vi "LiftMain.vi"(6 "Lift Override":bool, 8 "Error In":errorcluster, 9 "Reverse":bool, 10 "Forward":bool, 11 "Control Mode":enum16{"Open", "Control"}(ring)) -> (0 "Error Out":errorcluster, 2 "Switch Pressed":bool)   [LabVIEW 2016]
uses:
  <vilib>/Rock Robotics/SystemInterfaces/DIO/FPGA_DIORelayChannel.ctl
  <vilib>/Rock Robotics/WPI/Relay/WPI_RelayDirection.ctl
  <vilib>/Rock Robotics/SystemInterfaces/DIO/FPGA_DIOChannel.ctl
  <vilib>/Rock Robotics/WPI/Relay/WPI_RelayValue.ctl
  <vilib>/Rock Robotics/WPI/Switch/WPI_SwitchOpenLimit.vi
  <vilib>/Rock Robotics/Network Tables/NT Read Number.vi
panel:
  # "Lift Control Main VI\nFRC Team 34"
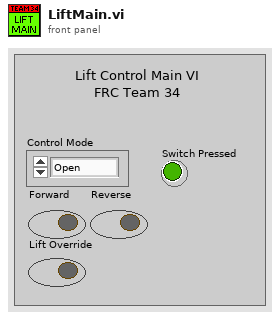
[diagram p1: front panel]
types:
  T1 = typedef "FPGA_DIOChannel.ctl" = enum8{"DIO 0", "DIO 1", "DIO 2", "DIO 3", "DIO 4", "DIO 5", "DIO 6", "DIO 7", "DIO 8", "DIO 9", "DIO MXP 0", "DIO MXP 1", "DIO MXP 2", "DIO MXP 3", "DIO MXP 4", "DIO MXP 5", "DIO MXP 6", "DIO MXP 7", "DIO MXP 8", "DIO MXP 9", "DIO MXP 10", "DIO MXP 11", "DIO MXP 12", "DIO MXP 13", "DIO MXP 14", "DIO MXP 15", "SPI Port CS1", "SPI Port CS2", "SPI Port CS3", "SPI Port MISO", "SPI Port MOSI", "Invalid"}
  T2 = typedef "WPI_RelayDirection.ctl" = enum16{"Both directions", "Forward only", "Reverse only"}
  T3 = typedef "FPGA_DIORelayChannel.ctl" = enum8{"Relay 0", "Relay 1", "Relay 2", "Relay 3", "Invalid"}
  T4 = typedef "WPI_RelayValue.ctl" = enum16{"Off", "On", "Forward", "Reverse"}
  T5 = typedef "WPI_SwitchDevRef.ctl" = cluster{"DevStatus":errorcluster, "DIO Channel":T1, "CntIndex":T6, "Normally Closed":bool}
  T6 = typedef "FPGA_CounterCtrSystemIndex.ctl" = enum8{"Ctr 0", "Ctr 1", "Ctr 2", "Ctr 3", "Ctr 4", "Ctr 5", "Ctr 6", "Ctr 7", "Invalid"}
  T7 = typedef "WPI_RelayDevRef.ctl" = cluster{"DevStatus":errorcluster, "Relay Channel":T3, "Relay Direction":T2}
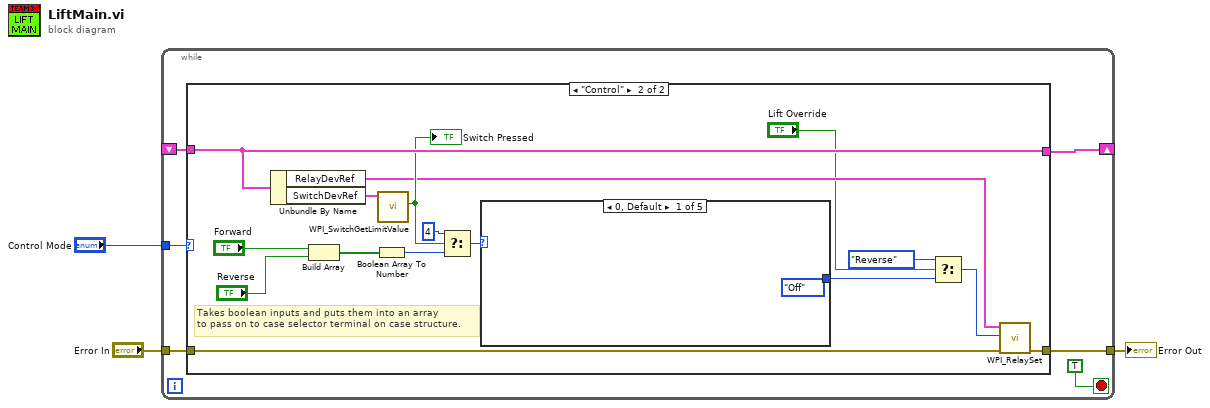
[diagram p0: block diagram]
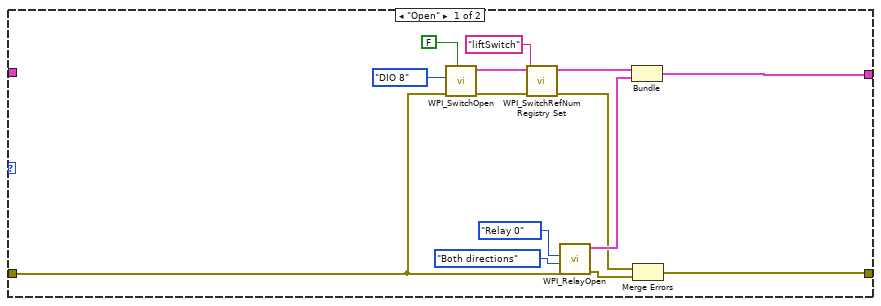
[diagram p2: hidden frame]
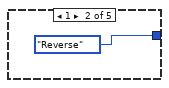
[diagram p3: hidden frame]
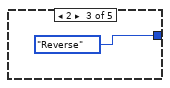
[diagram p4: hidden frame]
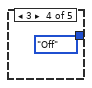
[diagram p5: hidden frame]
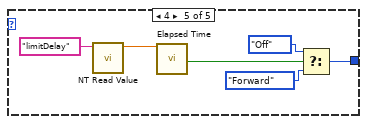
[diagram p6: hidden frame]
diagram:
  n1 = while {
    tunnel: "Control Mode" -> [w8]
    tunnel: "Error In" -> [w7]
    tunnel: [w6] -> w1
    shift-right: [w5] -> _
    shift-left: _ -> [w4]
    stop <- TRUE stop-if-true
    n2 = case shown="\"Control\"" w8 {
      tunnel: w7 -> [w17 w35]
      tunnel: [w15 w36] -> w6
      tunnel: [w19 w32] -> w5
      tunnel: w4 -> [_ w32]
      frame "Open" {
        n3 = call-poly <vilib>:"WPI_SwitchOpen.vi"("Normally Closed"=FALSE, "error in (no error)"=w17, "DIO Channel"=FPGA_DIOChannel."DIO 8") -> ("error out"=w13:errorcluster, "SwitchDevRef"=w14:T5)  [unwired: 7 in]
        n4 = call <vilib>:"WPI_SwitchRefNum Registry Set.vi"("error in (no error)"=w13, "refnum name"="liftSwitch", "SwitchDevRef"=w14) -> ("error out"=w11:errorcluster, "SwitchDevRef"=w12:T5)  [unwired: 7 in]
        n5 = call <vilib>:"WPI_RelayOpen.vi"("error in (no error)"=w17, "Relay Direction"=WPI_RelayDirection."Both directions", "Relay Channel"=FPGA_DIORelayChannel."Relay 0") -> ("error out"=w16:errorcluster, "RelayDevRef"=w20:T7)  [unwired: 7 in]
        n6 = Bundle("SwitchDevRef"=w12, "RelayDevRef"=w20) -> (w19:cluster{"SwitchDevRef":T5, "RelayDevRef":T7})  [unwired: 1 in]
        n7 = Merge Errors(w11, w16) -> (w15:errorcluster)
      }
      frame "Control" {
        # "Takes boolean inputs and puts them into an array\nto pass on to case selector terminal on case structure."
        n8 = Unbundle By Name(w32) -> ("RelayDevRef"=w28:T7, "SwitchDevRef"=w29:T5)
        n9 = Build Array("Forward", "Reverse") -> (w37:bool[])
        n10 = Boolean Array To Number(Boolean array=w37) -> (number=w33:u32)
        n11 = call <vilib>:"WPI_SwitchGetLimitValue.vi"("SwitchDevRef"=w29) -> ("Switch Pressed"=w31:bool)  [unwired: 8 in, 2 out]
        "Switch Pressed" <- w31
        n12 = Select(t=u32 4, s=w31, f=w33) -> (s? t:f=w34:u32)
        n13 = case shown="0, Default" w34 {
          tunnel: [WPI_RelayValue."Off" ("RelayValue") WPI_RelayValue."Reverse" ("RelayValue") WPI_RelayValue."Reverse" ("RelayValue") WPI_RelayValue."Off" ("RelayValue") w45] -> w27
          frame 0, Default {
          }
          frame 1 {
          }
          frame 2 {
          }
          frame 3 {
          }
          frame 4 {
            n14 = call-poly <vilib>:"NT Read Value.vi"("Name"="limitDelay") -> ("Numeric"=w48:dbl)  [unwired: 9 in, 1 out]
            n15 = call "Elapsed Time"("Time Target (s)"=w48) -> ("Time has Elapsed"=w47:bool)  [unwired: 11 in, 7 out]
            n16 = Select(t=WPI_RelayValue."Off" ("RelayValue"), s=w47, f=WPI_RelayValue."Forward") -> (s? t:f=w45:T4)
          }
        }
        n17 = Select(t=WPI_RelayValue."Reverse", s="Lift Override", f=w27) -> (s? t:f=w25:T4)
        n18 = call <vilib>:"WPI_RelaySet.vi"("error in (no error)"=w35, "RelayValue"=w25, "RelayDevRef"=w28) -> ("error out"=w36:errorcluster)  [unwired: 7 in, 1 out]
      }
    }
  }
  "Error Out" <- w1
